vi "Find User Events.vi"(7 "Config":refnum<class "TAF Proj Config.lvclass">, 8 "error in":errorcluster, 11 "VI References":refnum<vi>[](array[refnum])) -> (0 "error out":errorcluster, 3 "User Event  Info":T1[](array[typedef]))   [LabVIEW 2021, in "TAF Proj Document Type.lvlib" / "Project Parser.lvlib"]
uses:
  <vilib>/Wovalab/AntiDoc/Document Type/Add-ons/LabVIEW TAF Project/Project Parser/Project Parser.lvlib
  <vilib>/Wovalab/AntiDoc/Document Type/Add-ons/LabVIEW TAF Project/Project Parser/User Event Info.ctl
  <vilib>/Wovalab/AntiDoc/Document Type/Add-ons/LabVIEW TAF Project/TAF Proj Config/TAF Proj Config.lvclass
  <vilib>/Utility/traverseref.llb/TRef TravTarget.ctl
  <vilib>/Utility/traverseref.llb/VI Scripting - Traverse.lvlib
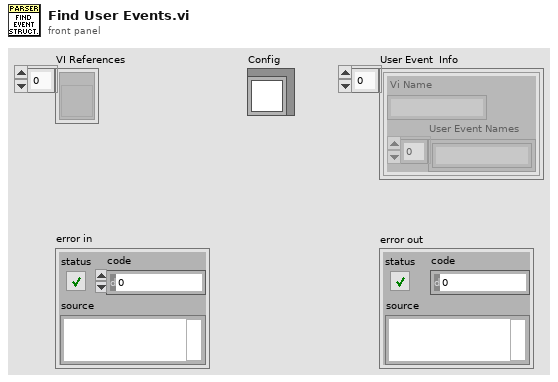
[diagram p1: front panel]
types:
  T1 = typedef "TAF Proj Document Type.lvlib/Project Parser.lvlib/User Event Info.ctl" = cluster{"Vi Name":string, "User Event Names":string[]}
  T2 = typedef "TRef TravTarget.ctl" = enum16{"FP", "BD", "Other"}
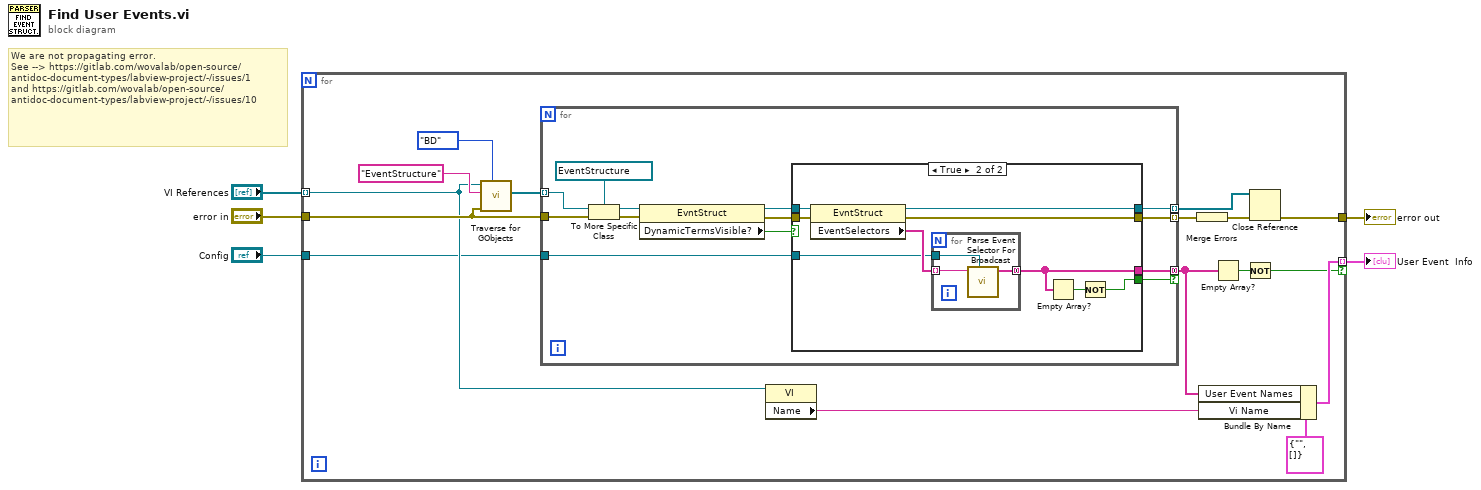
[diagram p0: block diagram]
diagram:
  # "We are not propagating error.\nSee --> https://gitlab.com/wovalab/open-source/antidoc-document-types/labview-project/-/issues/1\nand https://gitlab.com/wovalab/open-source/antidoc-document-types/labview-project/-/issues/10"
  n1 = for {
    tunnel: [w20] -> w5
    tunnel: "VI References" -> [w13] mode=indexing
    tunnel: [w11] -> w2 mode=indexing if=w9
    tunnel: "error in" -> [w19]
    tunnel: "Config" -> [w6]
    n2 = call <vilib>:"Traverse for GObjects.vi"("Traverse Target"=TRef_TravTarget."BD", "error in (no error)"=w19, "Class Name"="EventStructure", "VI Refnum"=w13) -> ("References"=w16:refnum<vi>[])  [unwired: 4 in, 3 out]
    n3 = for {
      tunnel: w16 -> [w30] mode=indexing
      tunnel: [w26] -> w12 mode=concatenating if=w25
      tunnel: w19 -> [w34]
      tunnel: [w31] -> w15 mode=indexing
      tunnel: [w23] -> w8 mode=indexing
      tunnel: w6 -> [w22]
      n4 = To More Specific Class(target class=refnum<vi> refnum ("reference"), reference=w30, error in=w34) -> (specific class reference=w29:refnum<vi>, error out=w33:errorcluster)
      n5 = property class="EvntStruct"(reference=w29, error in=w33) -> (reference out=w24:refnum<vi>, error out=w32:errorcluster, "DynamicTermsVisible?"=w27:bool)
      n6 = case shown="True" w27 {
        tunnel: [_ w40] -> w26
        tunnel: [_ w39] -> w25
        tunnel: w24 -> [w35 w43]
        tunnel: w32 -> [w36 w45]
        tunnel: [w36 w44] -> w31
        tunnel: [w35 w38] -> w23
        tunnel: w22 -> [_ w37]
        frame False {
        }
        frame True {
          n7 = property class="EvntStruct"(reference=w43, error in=w45) -> (reference out=w38:refnum<vi>, error out=w44:errorcluster, "EventSelectors"=w42:string[])
          n8 = for {
            tunnel: w42 -> [w48] mode=indexing
            tunnel: [w47] -> w40 mode=concatenating
            tunnel: w37 -> [w46]
            n9 = call <vilib>:"Parse Event Selector For Broadcast.vi"("Config"=w46, "Event Selector"=w48) -> ("Broadcast Events"=w47:string[])  [unwired: 9 in]
          }
          n10 = Empty Array?(array=w40) -> (empty?=w41:bool)
          n11 = Not(x=w41) -> (.not. x?=w39:bool)
        }
      }
    }
    n12 = property class="VI"(reference=w13) -> ("Name"=w7:string)  [unwired: 1 in, 2 out]
    n13 = Merge Errors(w15) -> (w21:errorcluster)
    n14 = Bundle By Name(cluster=T1 {"Vi Name"="", "User Event Names"=[]} ("User Event Info"), "User Event Names"=w12, "Vi Name"=w7) -> (w11:T1)
    n15 = Empty Array?(array=w12) -> (empty?=w10:bool)
    n16 = Not(x=w10) -> (.not. x?=w9:bool)
    n17 = Close Reference(reference=w8, error in (no error)=w21) -> (error out=w20:errorcluster)
  }
  "error out" <- w5
  "User Event  Info" <- w2
